vi "SimpleContainerStartedRegAndResolve.vi"() -> ()   [LabVIEW 2024, in "Module Container.lvlib"]
uses:
  Module Container.lvlib
  Module/RQMHModule.lvclass
  Scripting/templates/TemplateModule/TemplateModule.lvclass
panel:
  out "error out":errorcluster
  in  "stop":bool
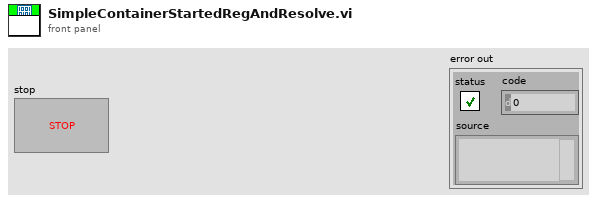
[diagram p1: front panel]
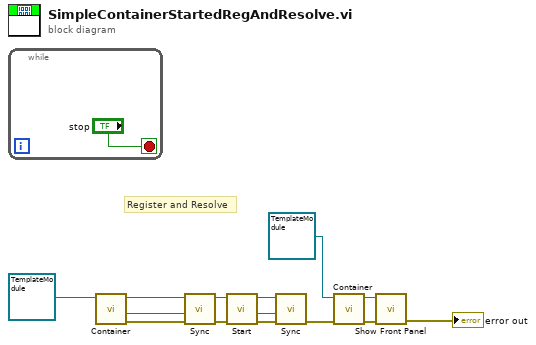
[diagram p0: block diagram]
diagram:
  # "Register and Resolve"
  n1 = while {
    stop <- "stop" stop-if-true
  }
  n2 = call "Container.vi"("Module Type"=refnum<class "TemplateModule.lvclass"> refnum ("TemplateModule.lvclass")) -> ("error out"=w6:errorcluster, "Handshake (if started)"=w4:refnum<class "RQMHStartup.lvclass">, "Module Instance"=w10:refnum<class "TemplateModule.lvclass">)  [unwired: 8 in]
  n3 = call "Sync.vi"("error in (no error)"=w6, "StartupHandshake out"=w4, "JQMHCore in"=w10) -> ("error out"=w1:errorcluster, "JQMHCore out"=w13:refnum<class "TemplateModule.lvclass">)  [unwired: 7 in]
  n4 = call "Start.vi"("error in (no error)"=w1, "JQMHCore in"=w13) -> ("error out"=w14:errorcluster, "StartupHandshake out"=w11:refnum<class "RQMHStartup.lvclass">, "JQMHCore out"=w12:refnum<class "TemplateModule.lvclass">)  [unwired: 7 in]
  n5 = call "Sync.vi"("error in (no error)"=w14, "StartupHandshake out"=w11, "JQMHCore in"=w12) -> ("error out"=w8:errorcluster)  [unwired: 7 in, 1 out]
  n6 = call "Container.vi"("error in (no error)"=w8, "Module Type"=refnum<class "TemplateModule.lvclass"> refnum ("TemplateModule.lvclass")) -> ("error out"=w3:errorcluster, "Module Instance"=w7:refnum<class "TemplateModule.lvclass">)  [unwired: 7 in, 1 out]
  n7 = call "Show Front Panel.vi"("error in (no error)"=w3, "JQMHCore in"=w7) -> ("error out"=→"error out":errorcluster)  [unwired: 8 in, 1 out]
